vi "VisionTest.vi"() -> ()   [LabVIEW 2019]
uses:
  <vilib>/Analysis/coordinate.llb/2D Cartesian Coordinate Shift (Array).vi
  <vilib>/Analysis/coordinate.llb/2D Cartesian Coordinate Rotation (Array).vi
  <vilib>/vision/NI_Vision_Development_Module.lvlib
  <vilib>/Analysis/NI_AALPro.lvlib
  KNRm_ReMi_OS6_436Motor.lvlibp
panel:
  out "100%?":bool
  in  "Range (Threshold 1)":cluster{"Lower value":sgl, "Upper value":sgl}={"Lower value"=0.0, "Upper value"=97.0}
  in  "BCG Values (Brightness 1)":T1={"Brightness"=14.920213, "Contrast"=75.893616, "Gamma"=0.54697555}
  in  "appended array":cluster{"X":dbl, "Y":dbl}[][](array[cluster])=[[{"X"=-47.53091149865394, "Y"=-51.61265055692628}, {"X"=-21.409316336691, "Y"=-52.40940259624713}, {"X"=7.531820971180464, "Y"=-50.24379818829546}, {"X"=34.723675975177635, "Y"=-49.29998044211228}, {"X"=62.50311529948201, "Y"=-48.069245788503636}], [{"X"=-52.10358780846479, "Y"=-23.573317003903952}, {"X"=-23.218349773016104, "Y"=-21.445937136105403}, {"X"=5.683945770158462, "Y"=-22.15858586504581}, {"X"=35.18585318767401, "Y"=-19.06306176014282}, {"X"=66.71847272117144, "Y"=-21.228561633901943}], [{"X"=-51.985118485666646, "Y"=6.629238139360316}, {"X"=-24.25833990412113, "Y"=12.579982375452046}, {"X"=5.656895686551195, "Y"=6.522155781007332}, {"X"=35.67862718864419, "Y"=7.798470020464374}, {"X"=69.44473388807687, "Y"=0.3684014734527225}], [{"X"=-54.7434454883762, "Y"=29.606207620157388}, {"X"=-24.38816628097914, "Y"=37.122414150924804}, {"X"=4.619057492645264, "Y"=32.696655394047305}, {"X"=35.01737200966194, "Y"=31.653332942710716}, {"X"=65.85863943682, "Y"=26.744342832725305}], [{"X"=-59.40958389987326, "Y"=69.68736705460744}, {"X"=-22.67716866450974, "Y"=68.0170935631974}, {"X"=9.882161579130868, "Y"=66.7477246147916}, {"X"=41.15360353471889, "Y"=62.8768714318752}, {"X"=71.97577084980611, "Y"=58.197728561186445}]]
  in  "appended array 3":cluster{dbl, dbl}[][](array[cluster])=[[{-50.0, -30.0}, {-20.0, -30.0}, {10.0, -30.0}, {40.0, -30.0}, {70.0, -30.0}], [{-50.0, 0.0}, {-20.0, 0.0}, {10.0, 0.0}, {40.0, 0.0}, {70.0, 0.0}], [{-50.0, 30.0}, {-20.0, 30.0}, {10.0, 30.0}, {40.0, 30.0}, {70.0, 30.0}], [{-50.0, 60.0}, {-20.0, 60.0}, {10.0, 60.0}, {40.0, 60.0}, {70.0, 60.0}], [{-50.0, 90.0}, {-20.0, 90.0}, {10.0, 90.0}, {40.0, 90.0}, {70.0, 90.0}]]
  out "Boolean array":bool[](array[boolean])
  out "y":dbl
  out "x":dbl
  out "stop":bool
  out "botton":bool
  in  "y":dbl=15.0 format="%#_13g"
  out "ColorDet Img":T2(plugin-control)
  out "G":u16
  out "B":u16
  out "Class":string
  out "output Brick (x, y, theta)":dbl[](array[numeric])
  in  "Grab":bool
  out "Particle Measurements (Real-World) (Particle Analysis 1)":dbl[][](array[numeric]) format="%.2f"
  out "Number of Matches":i32
  out "Cal Img":T2(plugin-control)
  out "Bin Img":T2(plugin-control)
  in  "Stop Button":bool
  # "r"
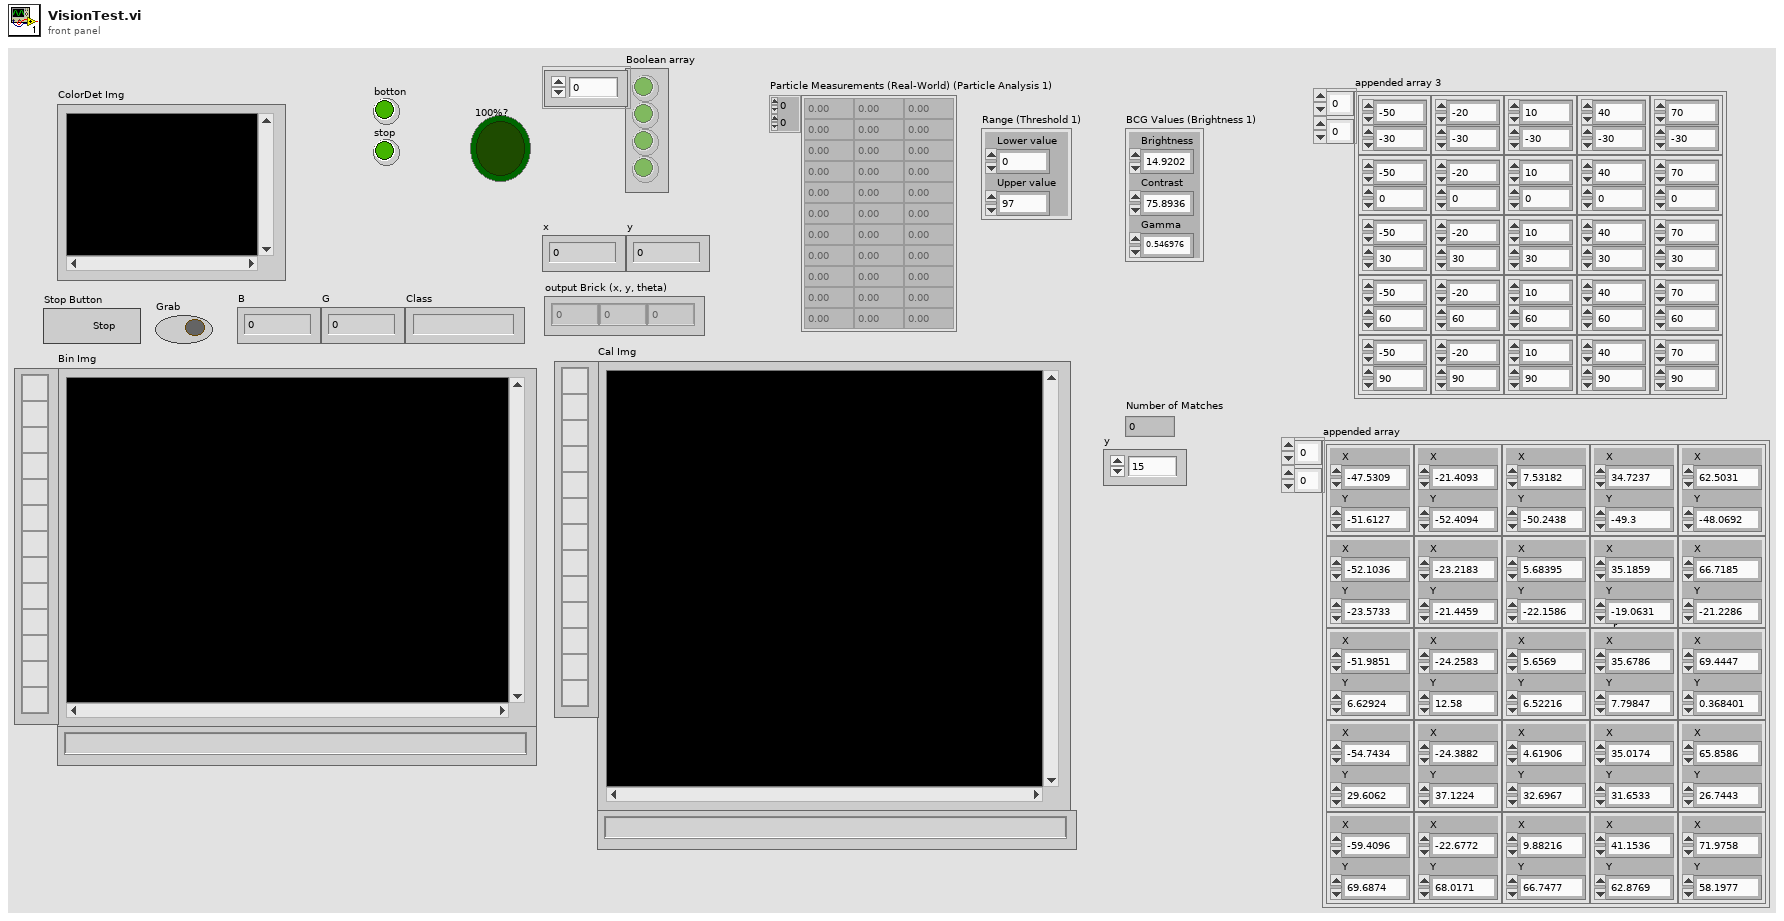
[diagram p1: front panel]
types:
  T1 = cluster{"Brightness":sgl, "Contrast":sgl, "Gamma":sgl}
  T2 = typedef "IMAQ Image.ctl" = refnum<image>
  T3 = typedef "Image Type" = u32
  T4 = cluster{"Interpolation Type":enum32{"Zero Order", "Bilinear", "Quadratic", "Cubic", "Bilinear Fixed"}, "Destination Width":u32, "Destination Height":u32, "Fill Value":sgl}
  T5 = cluster{"Particle Measurements (Real-World) (Particle Analysis 1)":dbl[], "Class":string}
  T6 = enum16{"P1", "P2", "P3", "P4", "P5", "P6", "OUT", "take a picture"}
  T7 = cluster{"Numeric":u8, "Numeric":u8, "Numeric":u8, "Numeric":u8}
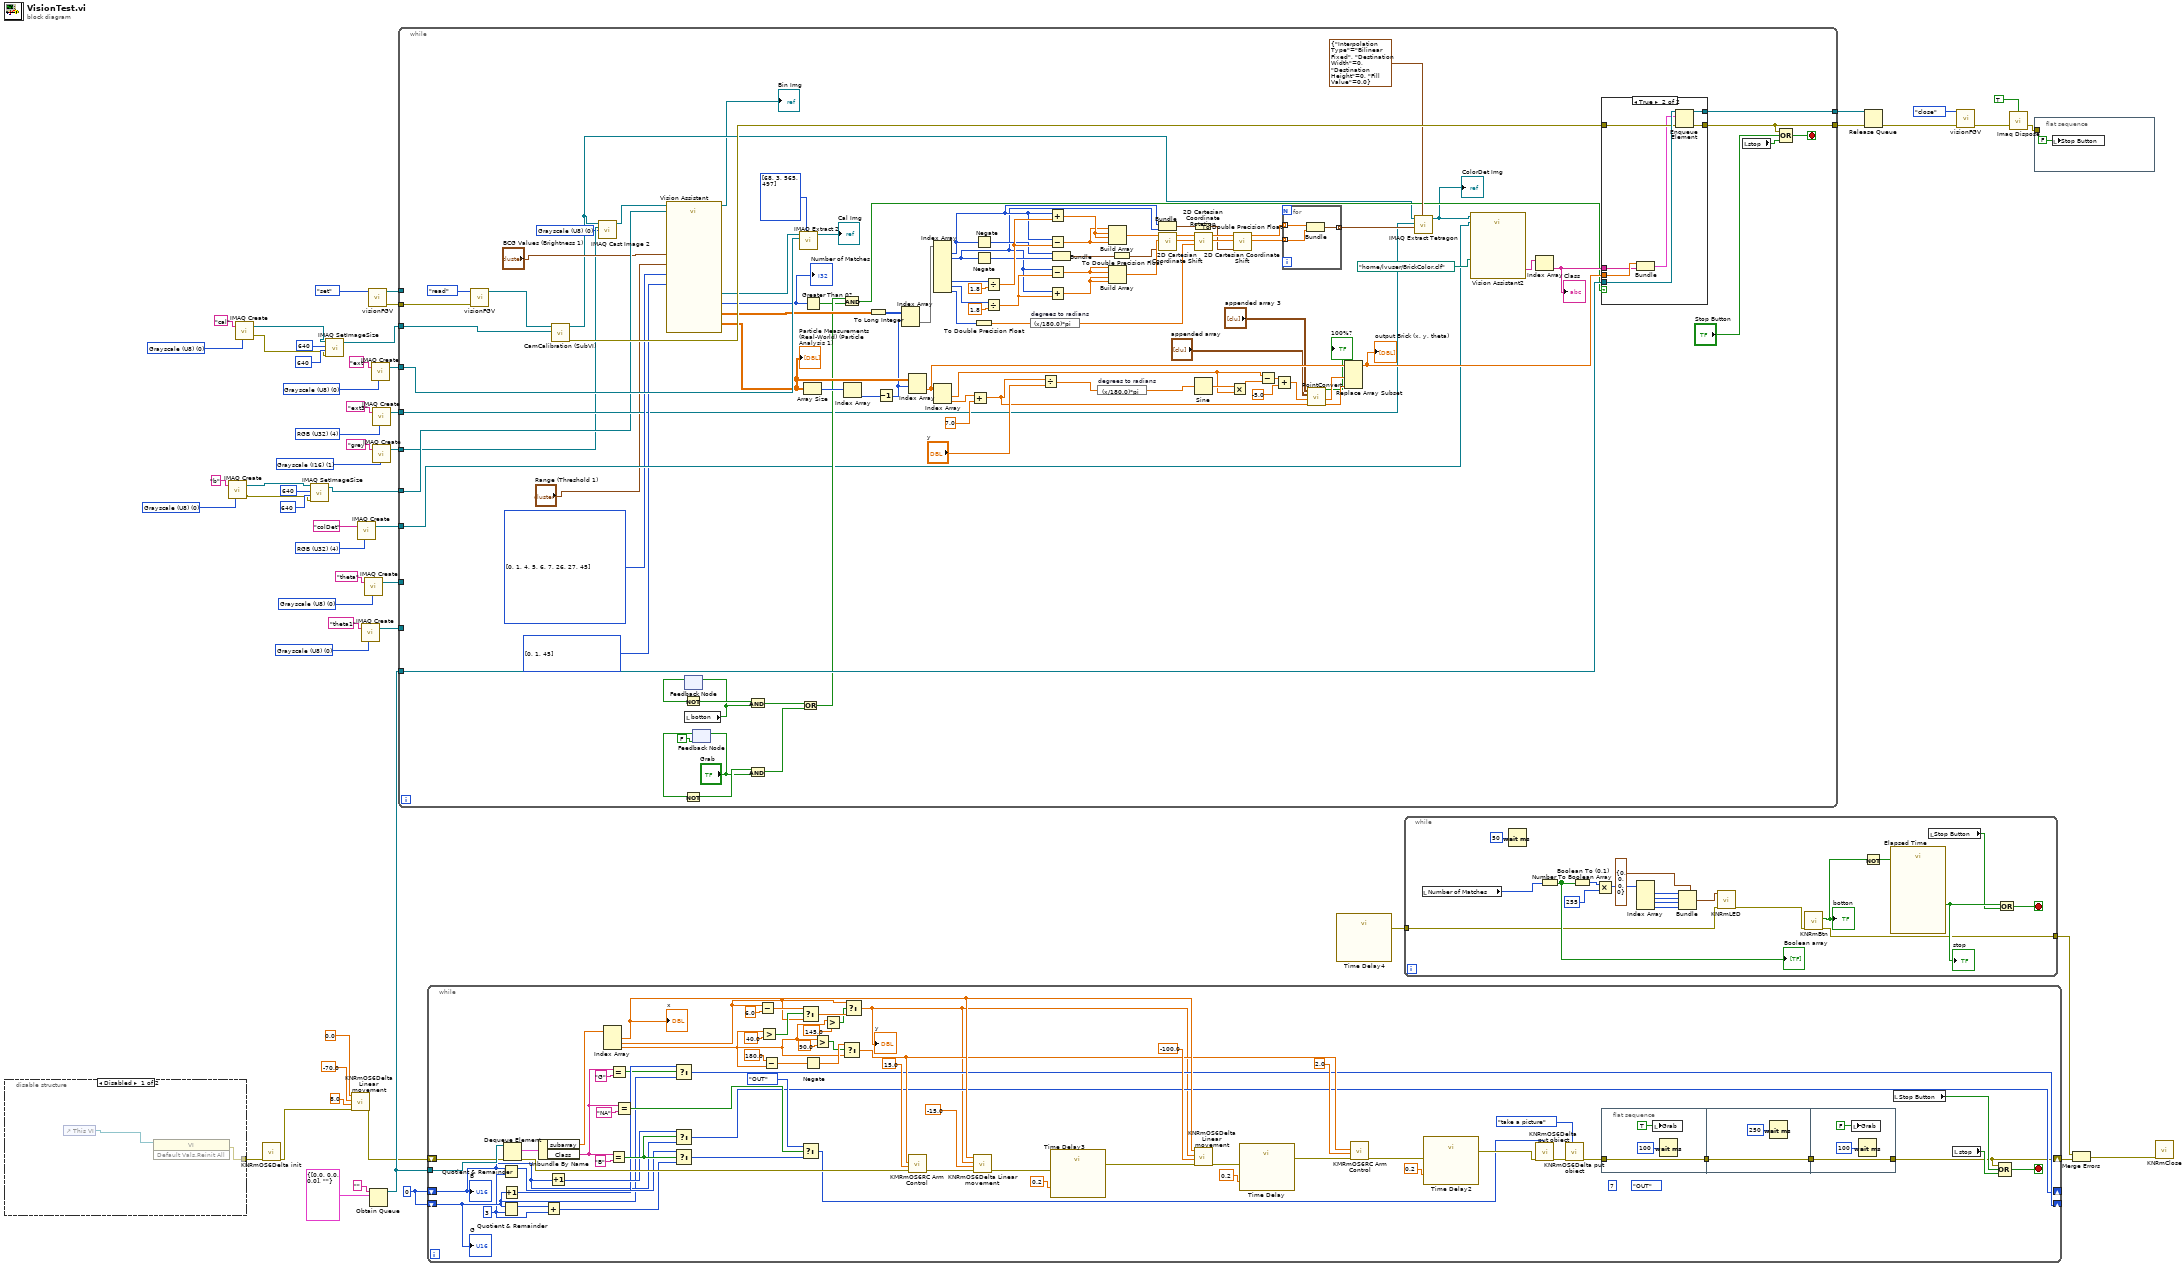
[diagram p0: block diagram]
diagram:
  w14 = T3 0 items=["Grayscale (U8)", "Grayscale (I16)", "Grayscale (SGL)", "Complex (CSG)", "RGB (U32)", "HSL (U32)", "RGB (U64)", "Grayscale (U16)"] ("Image Type")
  w24 = T3 0 items=["Grayscale (U8)", "Grayscale (I16)", "Grayscale (SGL)", "Complex (CSG)", "RGB (U32)", "HSL (U32)", "RGB (U64)", "Grayscale (U16)"] ("Image Type")
  w29 = T3 4 items=["Grayscale (U8)", "Grayscale (I16)", "Grayscale (SGL)", "Complex (CSG)", "RGB (U32)", "HSL (U32)", "RGB (U64)", "Grayscale (U16)"] ("Image Type")
  w31 = u16 0
  w34 = T3 4 items=["Grayscale (U8)", "Grayscale (I16)", "Grayscale (SGL)", "Complex (CSG)", "RGB (U32)", "HSL (U32)", "RGB (U64)", "Grayscale (U16)"] ("Image Type")
  w42 = T3 0 items=["Grayscale (U8)", "Grayscale (I16)", "Grayscale (SGL)", "Complex (CSG)", "RGB (U32)", "HSL (U32)", "RGB (U64)", "Grayscale (U16)"] ("Image Type")
  w45 = T3 0 items=["Grayscale (U8)", "Grayscale (I16)", "Grayscale (SGL)", "Complex (CSG)", "RGB (U32)", "HSL (U32)", "RGB (U64)", "Grayscale (U16)"] ("Image Type")
  w47 = T3 0 items=["Grayscale (U8)", "Grayscale (I16)", "Grayscale (SGL)", "Complex (CSG)", "RGB (U32)", "HSL (U32)", "RGB (U64)", "Grayscale (U16)"] ("Image Type")
  w49 = T3 1 items=["Grayscale (U8)", "Grayscale (I16)", "Grayscale (SGL)", "Complex (CSG)", "RGB (U32)", "HSL (U32)", "RGB (U64)", "Grayscale (U16)"] ("Image Type")
  n1 = disable-structure shown="Disabled" {
    disable-tunnel: [w57 _] -> w12
    frame Disabled {
      n2 = control-ref of="This VI"() -> (w58:refnum<vi>)
      n3 = invoke class="VI" method="Default Vals.Reinit All"(reference=w58) -> (error out=w57:errorcluster)  [unwired: 2 in, 2 out]
    }
    frame Enabled {
    }
  }
  n4 = call "IMAQ Create"("Image Name"="b", "Image Type"=w42) -> ("New Image"=w3:T2, "error out"=w2:errorcluster)  [unwired: 3 in]
  n5 = call "IMAQ Create"("Image Name"="cal", "Image Type"=w47) -> ("New Image"=w8:T2, "error out"=w7:errorcluster)  [unwired: 3 in]
  n6 = call "KNRmOS6Delta init.vi"("error in (no error)"=w12) -> ("error out"=w17:errorcluster)  [unwired: 10 in]
  n7 = call "IMAQ SetImageSize"("error in (no error)"=w2, "Y Resolution"=640, "X Resolution"=640, "Image"=w3) -> ("Image Out"=w1:T2)  [unwired: 1 in, 1 out]
  n8 = call "IMAQ SetImageSize"("error in (no error)"=w7, "Y Resolution"=640, "X Resolution"=640, "Image"=w8) -> ("Image Out"=w6:T2)  [unwired: 1 in, 1 out]
  n9 = call "KNRmOS6Delta Linear movement.vi"("error in (no error)"=w17, "z0"=8.0, "y0"=-70.0, "x0"=0.0) -> ("error out"=w16:errorcluster)  [unwired: 7 in]
  n10 = call "IMAQ Create"("Image Name"="colDet", "Image Type"=w34) -> ("New Image"=w33:T2)  [unwired: 3 in, 1 out]
  n11 = call "IMAQ Create"("Image Name"="theta1", "Image Type"=w14) -> ("New Image"=w13:T2)  [unwired: 3 in, 1 out]
  n12 = call "IMAQ Create"("Image Name"="theta", "Image Type"=w24) -> ("New Image"=w22:T2)  [unwired: 3 in, 1 out]
  n13 = call "visionFGV.vi"("Function"=enum16{"set", "read", "close"}."set") -> ("error out"=w51:errorcluster, "Image Out fgv"=w55:T2)  [unwired: 9 in]
  n14 = Obtain Queue(name (unnamed)="", element data type=cluster{"subarray":dbl[], "Class":string} {"subarray"=[0.0, 0.0, 0.0], "Class"=""}) -> (queue out=w39:refnum<queue>)  [unwired: 3 in, 2 out]
  n15 = call "IMAQ Create"("Image Name"="ext", "Image Type"=w45) -> ("New Image"=w44:T2)  [unwired: 3 in, 1 out]
  n16 = call "IMAQ Create"("Image Name"="ext3", "Image Type"=w29) -> ("New Image"=w28:T2)  [unwired: 3 in, 1 out]
  n17 = call "IMAQ Create"("Image Name"="grey", "Image Type"=w49) -> ("New Image"=w48:T2)  [unwired: 3 in, 1 out]
  n18 = while {
    tunnel: w55 -> [_]
    tunnel: w51 -> [w158]
    tunnel: w48 -> [w64]
    tunnel: w6 -> [w75]
    tunnel: w44 -> [w156]
    tunnel: w1 -> [w74]
    tunnel: w39 -> [w154]
    tunnel: [w98] -> w38
    tunnel: [w152] -> w36
    tunnel: w33 -> [w87]
    tunnel: w28 -> [w78]
    tunnel: w22 -> [_]
    tunnel: w13 -> [_]
    stop <- w95 stop-if-true
    w62 = T3 0 items=["Grayscale (U8)", "Grayscale (I16)", "Grayscale (SGL)", "Complex (CSG)", "RGB (U32)", "HSL (U32)", "RGB (U64)", "Grayscale (U16)"] ("Image Type")
    w81 = i32[] [0, 1, 4, 5, 6, 7, 26, 27, 45] items=["Center of Mass X", "Center of Mass Y", "First Pixel X", "First Pixel Y", "Bounding Rect Left", "Bounding Rect Top", "Bounding Rect Right", "Bounding Rect Bottom", "Max Feret Diameter Start X", "Max Feret Diameter Start Y", "Max Feret Diameter End X", "Max Feret Diameter End Y", "Max Horiz. Segment Length Left", "Max Horiz. Segment Length Right", "Max Horiz. Segment Length Row", "-", "Bounding Rect Width", "Bounding Rect Height", "Bounding Rect Diagonal", "Perimeter", "Convex Hull Perimeter", "Holes' Perimeter", "Max Feret Diameter", "Equivalent Ellipse Major Axis", "Equivalent Ellipse Minor Axis", "Equivalent Ellipse Minor Axis (Feret)", "Equivalent Rect Long Side", "Equivalent Rect Short Side", "Equivalent Rect Diagonal", "Equivalent Rect Short Side (Feret)", "Average Horiz. Segment Length", "Average Vert. Segment Length", "Hydraulic Radius", "Waddel Disk Diameter", "-", "Area", "Holes' Area", "Particle & Holes' Area", "Convex Hull Area", "Image Area", "-", "Number of Holes", "Number of Horiz. Segments", "Number of Vert. Segments", "-", "Orientation", "Max Feret Diameter Orientation", "-", "% Area/Image Area", "% Area/(Particle & Holes' Area)", "Ratio of Equivalent Ellipse Axes", "Ratio of Equivalent Rect Sides", "-", "Elongation Factor", "Compactness Factor", "Heywood Circularity Factor", "Type Factor", "-", "Sum X", "Sum Y", "Sum XX", "Sum XY", "Sum YY", "Sum XXX", "Sum XXY", "Sum XYY", "Sum YYY", "-", "Moment of Inertia XX", "Moment of Inertia XY", "Moment of Inertia YY", "Moment of Inertia XXX", "Moment of Inertia XXY", "Moment of Inertia XYY", "Moment of Inertia YYY", "Norm. Moment of Inertia XX", "Norm. Moment of Inertia XY", "Norm. Moment of Inertia YY", "Norm. Moment of Inertia XXX", "Norm. Moment of Inertia XXY", "Norm. Moment of Inertia XYY", "Norm. Moment of Inertia YYY", "Hu Moment 1", "Hu Moment 2", "Hu Moment 3", "Hu Moment 4", "Hu Moment 5", "Hu Moment 6", "Hu Moment 7"] ("Pixel Measurements (Particle Analysis 1)")
    w80 = i32[] [0, 1, 45] items=["Center of Mass X", "Center of Mass Y", "First Pixel X", "First Pixel Y", "Bounding Rect Left", "Bounding Rect Top", "Bounding Rect Right", "Bounding Rect Bottom", "Max Feret Diameter Start X", "Max Feret Diameter Start Y", "Max Feret Diameter End X", "Max Feret Diameter End Y", "Max Horiz. Segment Length Left", "Max Horiz. Segment Length Right", "Max Horiz. Segment Length Row", "-", "Bounding Rect Width", "Bounding Rect Height", "Bounding Rect Diagonal", "Perimeter", "Convex Hull Perimeter", "Holes' Perimeter", "Max Feret Diameter", "Equivalent Ellipse Major Axis", "Equivalent Ellipse Minor Axis", "Equivalent Ellipse Minor Axis (Feret)", "Equivalent Rect Long Side", "Equivalent Rect Short Side", "Equivalent Rect Diagonal", "Equivalent Rect Short Side (Feret)", "Average Horiz. Segment Length", "Average Vert. Segment Length", "Hydraulic Radius", "Waddel Disk Diameter", "-", "Area", "Holes' Area", "Particle & Holes' Area", "Convex Hull Area", "Image Area", "-", "Number of Holes", "Number of Horiz. Segments", "Number of Vert. Segments", "-", "Orientation", "Max Feret Diameter Orientation", "-", "% Area/Image Area", "% Area/(Particle & Holes' Area)", "Ratio of Equivalent Ellipse Axes", "Ratio of Equivalent Rect Sides", "-", "Elongation Factor", "Compactness Factor", "Heywood Circularity Factor", "Type Factor", "-", "Sum X", "Sum Y", "Sum XX", "Sum XY", "Sum YY", "Sum XXX", "Sum XXY", "Sum XYY", "Sum YYY", "-", "Moment of Inertia XX", "Moment of Inertia XY", "Moment of Inertia YY", "Moment of Inertia XXX", "Moment of Inertia XXY", "Moment of Inertia XYY", "Moment of Inertia YYY", "Norm. Moment of Inertia XX", "Norm. Moment of Inertia XY", "Norm. Moment of Inertia YY", "Norm. Moment of Inertia XXX", "Norm. Moment of Inertia XXY", "Norm. Moment of Inertia XYY", "Norm. Moment of Inertia YYY", "Hu Moment 1", "Hu Moment 2", "Hu Moment 3", "Hu Moment 4", "Hu Moment 5", "Hu Moment 6", "Hu Moment 7"] ("Real-World Measurements (Particle Analysis 1)")
    n19 = call "visionFGV.vi"("Error In"=w158, "Function"=enum16{"set", "read", "close"}."read") -> ("Image Out fgv"=w77:T2)  [unwired: 8 in, 1 out]
    n20 = call "CamCalibration (SubVI).vi"("Image Dst"=w75, "Image In"=w77) -> ("error out"=w153:errorcluster, "Image Out"=w63:T2)  [unwired: 8 in]
    n21 = call "IMAQ Cast Image 2"("Image Src"=w63, "Image Dst"=w64, "Image Type"=w62) -> ("Image Dst Out"=w61:T2)  [unwired: 11 in, 1 out]
    n22 = call "Vision Assistant"("Image In"=w61, "Image Dst"=w74, "BCG Values (Brightness 1)"="BCG Values (Brightness 1)", "Range (Threshold 1)"="Range (Threshold 1)", "Pixel Measurements (Particle Analysis 1)"=w81, "Real-World Measurements (Particle Analysis 1)"=w80) -> ("Image Out"=→"Bin Img":T2, "Number of Particles (Particle Analysis 1)"=w101:i32, "Particle Measurements (Real-World) (Particle Analysis 1)"=w147:dbl[][], "Particle Measurements (Pixels) (Particle Analysis 1)"=w139:dbl[][], "Image Buffer (Image Buffer 2)"=w145:T2)  [unwired: 16 in, 1 out]
    "Number of Matches" <- w101
    "Particle Measurements (Real-World) (Particle Analysis 1)" <- w147
    n23 = feedback #1() -> (w93:bool)  [unwired: 1 in]
    n24 = Not(x=w93) -> (.not. x?=w92:bool)
    n25 = local read "botton"() -> (w91:bool)
    n26 = feedback-in #1(w91) -> ()
    n27 = feedback-in #2("Grab") -> ()
    n28 = feedback #2(FALSE ("Grab")) -> (w151:bool)
    n29 = Not(x=w151) -> (.not. x?=w150:bool)
    n30 = And(x=w92, y=w91) -> (x .and. y?=w90:bool)
    n31 = And(x=w150, y="Grab") -> (x .and. y?=w103:bool)
    n32 = call "IMAQ Extract 2"("Optional Rectangle"=i32[] [68, 3, 565, 497] ("Global Rectangle"), "Image Dst"=w156, "Image Src"=w145) -> ("Image Dst Out"=→"Cal Img":T2)  [unwired: 7 in, 1 out]
    n33 = Or(x=w90, y=w103) -> (x .or. y?=w102:bool)
    n34 = Array Size(array=w147) -> (size(s)=w148:i32[])
    n35 = Greater Than 0?(x=w101) -> (x > 0?=w100:bool)
    n36 = And(x=w102, y=w100) -> (x .and. y?=w99:bool)
    n37 = Index Array(array=w148) -> (element=w146:i32)  [unwired: 1 in]
    n38 = To Long Integer(number=w139) -> (32bit integer=w138:i32[][])
    n39 = Decrement(x=w146) -> (x-1=w79:i32)
    n40 = Index Array(array=w138, index (row)=w79) -> (element=w76:i32[])  [unwired: 1 in]
    n41 = Index Array(array=w147, index (row)=w79) -> (element=w141:dbl[])  [unwired: 1 in]
    n42 = Index Array(array=w76) -> (element #1=w119:i32, element #2=w118:i32, element #7=w129:i32, element #8=w125:i32, element #9=w132:i32)  [unwired: 9 in, 4 out]
    n43 = Index Array(array=w141) -> (element #1=w69:dbl, element #2=w83:dbl)  [unwired: 2 in]
    n44 = Add(x=w83, y=7.0) -> (x+y=w73:dbl)
    n45 = Negate(x=w119) -> (-x=w121:i32)
    n46 = Negate(x=w118) -> (-x=w122:i32)
    n47 = To Double Precision Float(number=w132) -> (double precision float=w123:dbl)
    n48 = Divide(x=w129, y=1.8) -> (x/y=w127:dbl)
    n49 = Divide(x=w125, y=1.8) -> (x/y=w124:dbl)
    n50 = expression code="(x/180.0)*pi" "degrees to radians"(w123) -> (w131:dbl)
    n51 = Divide(x=w73, y="y") -> (x/y=w143:dbl)
    n52 = Add(x=w119, y=w127) -> (x+y=w136:dbl)
    n53 = Subtract(x=w119, y=w127) -> (x-y=w135:dbl)
    n54 = Subtract(x=w118, y=w124) -> (x-y=w134:dbl)
    n55 = Add(x=w118, y=w124) -> (x+y=w133:dbl)
    n56 = Bundle(w121, w122) -> (w120:cluster{i32, i32})  [unwired: 1 in]
    n57 = expression code="(x/180.0)*pi" "degrees to radians"(w143) -> (w108:dbl)
    n58 = Build Array(w135, w136, w136, w135) -> (w117:dbl[])
    n59 = Build Array(w134, w134, w133, w133) -> (w116:dbl[])
    n60 = To Double Precision Float(number=w120) -> (double precision float=w106:cluster{dbl, dbl})
    n61 = Bundle("Numeric"=w119, "Numeric"=w118) -> (w111:cluster{"Numeric":i32, "Numeric":i32})  [unwired: 1 in]
    n62 = call-poly <vilib>:"2D Cartesian Coordinate Shift.vi"("shift"=w106, "Y"=w116, "X"=w117) -> ("Y Out"=w114:dbl[], "X Out"=w115:dbl[])  [unwired: 6 in, 1 out]
    n63 = To Double Precision Float(number=w111) -> (double precision float=w107:cluster{"Numeric":dbl, "Numeric":dbl})
    n64 = call-poly <vilib>:"2D Cartesian Coordinate Rotation.vi"("theta"=w131, "Y"=w114, "X"=w115) -> ("Y Out"=w112:dbl[], "X Out"=w113:dbl[])  [unwired: 6 in, 1 out]
    n65 = Sine(x=w108) -> (sin(x)=w105:dbl)
    n66 = Multiply(x=w105, y=w69) -> (x*y=w142:dbl)
    n67 = call-poly <vilib>:"2D Cartesian Coordinate Shift.vi"("shift"=w107, "Y"=w112, "X"=w113) -> ("Y Out"=w109:dbl[], "X Out"=w110:dbl[])  [unwired: 6 in, 1 out]
    n68 = Subtract(x=w69, y=w142) -> (x-y=w85:dbl)
    n69 = Add(x=w85, y=-5.0) -> (x+y=w70:dbl)
    n70 = for {
      tunnel: w110 -> [w162] mode=indexing
      tunnel: w109 -> [w161] mode=indexing
      tunnel: [w160] -> w130 mode=indexing
      n71 = Bundle("Numeric"=w162, "Numeric"=w161) -> (w160:cluster{"Numeric":dbl, "Numeric":dbl})  [unwired: 1 in]
    }
    n72 = call "PointConvert.vi"("RealWorldY"=w73, "RealWorldX"=w70, "RealWorldXY"="appended array", "DeltaXY"="appended array 3") -> ("DeltaY"=w71:dbl, "DeltaX"=w72:dbl, "100%?"=→"100%?":bool)  [unwired: 5 in]
    n73 = Replace Array Subset(array=w141, new element #1=w72, new element #2=w71) -> (w140:dbl[])  [unwired: 2 in]
    "output Brick (x, y, theta)" <- w140
    n74 = call-poly "IMAQ Extract Tetragon"("Options"=T4 {"Interpolation Type"=enum."Bilinear Fixed", "Destination Width"=0, "Destination Height"=0, "Fill Value"=0.0}, "Tetragon"=w130, "Image Dst"=w78, "Image Src"=w63) -> ("Image Dst Out"=w88:T2)  [unwired: 6 in, 1 out]
    "ColorDet Img" <- w88
    n75 = call "Vision Assistant2"("Image In"=w88, "Image Dst"=w87, "File Path (Color Classification 1)"=path "/home/lvuser/BrickColor.clf") -> ("Classes (Color Classification 1)"=w86:string[])  [unwired: 22 in, 2 out]
    n76 = Index Array(array=w86) -> (element=w104:string)  [unwired: 1 in]
    "Class" <- w104
    n77 = case shown="True" w99 {
      tunnel: w154 -> [w163 w171]
      tunnel: w140 -> [_ w167]
      tunnel: [w164 w170] -> w98
      tunnel: w153 -> [w164 w169]
      tunnel: [w163 w168] -> w152
      tunnel: w104 -> [_ w166]
      frame False {
      }
      frame True {
        n78 = Bundle("Particle Measurements (Real-World) (Particle Analysis 1)"=w167, "Class"=w166) -> (w165:T5)  [unwired: 1 in]
        n79 = Enqueue Element(queue=w171, element=w165, error in (no error)=w169) -> (queue out=w168:refnum<queue>, error out=w170:errorcluster)  [unwired: 1 in, 1 out]
      }
    }
    n80 = local read "stop"() -> (w96:bool)
    n81 = Compound Arithmetic op=OR(w98, "Stop Button", w96) -> (w95:bool)
  }
  n82 = while {
    tunnel: w39 -> [w236]
    shift-right: [w177] -> w26
    shift-left: w16 -> [w228]
    shift-right: [w200] -> _
    shift-left: w31 -> [w199]
    shift-right: [w201] -> _
    shift-left: w31 -> [w198]
    stop <- w182 stop-if-true
    w196 = u16 3 ("y")
    (unwired) T6."OUT" ("move to")
    (unwired) 7 ("y")
    n83 = Quotient & Remainder(x=w199, y=w196) -> (x-y*floor(x/y)=w206:u16)  [unwired: 1 out]
    n84 = Increment(x=w198) -> (x+1=w205:u16)
    n85 = Quotient & Remainder(x=w198, y=w196) -> (x-y*floor(x/y)=w197:u16)  [unwired: 1 out]
    n86 = Dequeue Element(queue=w236, error in (no error)=w228) -> (element=w214:cluster{"subarray":dbl[], "Class":string}, error out=w232:errorcluster)  [unwired: 1 in, 2 out]
    n87 = Unbundle By Name(w214) -> ("subarray"=w213:dbl[], "Class"=w203:string)
    n88 = Add(x=w197, y=w196) -> (x+y=w195:u16)
    n89 = Increment(x=w199) -> (x+1=w207:u16)
    n90 = Index Array(array=w213) -> (element #1=w223:dbl, element #2=w185:dbl, element #3=w174:dbl)  [unwired: 3 in]
    "x" <- w223
    n91 = Equal?(x=w203, y="B") -> (x = y?=w208:bool)
    n92 = Equal?(x=w203, y="G") -> (x = y?=w202:bool)
    n93 = Equal?(x=w203, y="NA") -> (x = y?=w211:bool)
    n94 = Select(t=w205, s=w202, f=w198) -> (s? t:f=w201:u16)
    n95 = Select(t=w207, s=w208, f=w199) -> (s? t:f=w200:u16)
    n96 = Select(t=w206, s=w208, f=w195) -> (s? t:f=w194:u16)
    n97 = Subtract(x=w185, y=6.0 ("y 2")) -> (x-y=w187:dbl)
    n98 = Greater?(x=w174, y=40.0) -> (0:w188:bool)
    n99 = Subtract(x=180.0, y=w174) -> (x-y=w216:dbl)
    n100 = Select(t=w187, s=w188, f=w185) -> (s? t:f=w186:dbl)
    n101 = Select(t=T6."OUT" ("move to"), s=w211, f=w194) -> (s? t:f=w193:u16)
    n102 = Negate(x=w216) -> (-x=w215:dbl)
    n103 = Greater?(x=w174, y=90.0) -> (0:w192:bool)
    n104 = Greater?(x=w174, y=145.0) -> (0:w172:bool)
    n105 = Select(t=w215, s=w192, f=w174) -> (s? t:f=w217:dbl)
    n106 = Select(t=w185, s=w172, f=w186) -> (s? t:f=w190:dbl)
    "y" <- w190
    n107 = call "KMRmOS6RC Arm Control.vi"("error in (no error)"=w232, "clip"=15.0, "turn"=w217) -> ("error out"=w233:errorcluster)  [unwired: 6 in, 2 out]
    n108 = call "KNRmOS6Delta Linear movement.vi"("error in (no error)"=w233, "z0"=-15.0, "y0"=w190, "x0"=w223) -> ("error out"=w181:errorcluster)  [unwired: 7 in]
    n109 = call "Time Delay3"("error in (no error)"=w181, "Delay Time (s)"=0.2) -> ("error out"=w179:errorcluster)  [unwired: 9 in]
    n110 = call "KNRmOS6Delta Linear movement.vi"("error in (no error)"=w179, "z0"=-100.0, "y0"=w190, "x0"=w223) -> ("error out"=w224:errorcluster)  [unwired: 7 in]
    n111 = call "Time Delay"("error in (no error)"=w224, "Delay Time (s)"=0.2) -> ("error out"=w226:errorcluster)  [unwired: 9 in]
    n112 = call "KMRmOS6RC Arm Control.vi"("error in (no error)"=w226, "clip"=2.0, "turn"=w217) -> ("error out"=w222:errorcluster)  [unwired: 6 in, 2 out]
    n113 = call "Time Delay2"("error in (no error)"=w222, "Delay Time (s)"=0.2) -> ("error out"=w221:errorcluster)  [unwired: 9 in]
    n114 = call "KNRmOS6Delta put obiect.vi"("move to"=w193, "error in (no error)"=w221) -> ("error in (no error) 2"=w230:errorcluster)  [unwired: 9 in]
    n115 = call "KNRmOS6Delta put obiect.vi"("move to"=T6."take a picture", "error in (no error)"=w230) -> ("error in (no error) 2"=w178:errorcluster)  [unwired: 9 in]
    n116 = flat-sequence {
      tunnel: w178 -> [w239]
      tunnel: [w239] -> w175
      tunnel: [w240] -> w176
      tunnel: w175 -> [w240]
      tunnel: [w243] -> w177
      tunnel: w176 -> [w243]
      frame #0 {
        n117 = local write "Grab"(TRUE ("Grab")) -> ()
        n118 = Wait (ms)(milliseconds to wait=u32 100) -> ()  [unwired: 1 out]
      }
      frame #1 {
        n119 = Wait (ms)(milliseconds to wait=u32 250) -> ()  [unwired: 1 out]
      }
      frame #2 {
        n120 = local write "Grab"(FALSE ("Grab")) -> ()
        n121 = Wait (ms)(milliseconds to wait=u32 100) -> ()  [unwired: 1 out]
      }
    }
    n122 = local read "Stop Button"() -> (w184:bool)
    n123 = local read "stop"() -> (w183:bool)
    n124 = Compound Arithmetic op=OR(w177, w184, w183) -> (w182:bool)
    "B" <- w199
    "G" <- w198
  }
  n125 = call "Time Delay4"() -> ("error out"=w25:errorcluster)  [unwired: 11 in]
  n126 = while {
    tunnel: [w259] -> w27
    tunnel: w25 -> [w245]
    stop <- w262 stop-if-true
    n127 = local read "Number of Matches"() -> (w247:i32)
    n128 = Wait (ms)(milliseconds to wait=u32 50) -> ()  [unwired: 1 out]
    n129 = Number To Boolean Array(number=w247) -> (Boolean array=w246:bool[])
    "Boolean array" <- w246
    n130 = Boolean To (0,1)(Boolean=w246) -> (0, 1=w255:i16[])
    n131 = Multiply(x=w255, y=255) -> (x*y=w254:i32[])
    n132 = Index Array(array=w254) -> (element #1=w252:i32, element #2=w251:i32, element #3=w250:i32, element #4=w249:i32)  [unwired: 4 in]
    n133 = Bundle(cluster=T7 {"Numeric"=0, "Numeric"=0, "Numeric"=0, "Numeric"=0} ("LEDSet"), "Numeric"=w252, "Numeric"=w251, "Numeric"=w250, "Numeric"=w249) -> (w256:T7)
    n134 = call "KNRmLED.vi"("error in"=w245, "LEDSet"=w256) -> ("error out"=w248:errorcluster)  [unwired: 9 in]
    n135 = call "KNRmBtn.vi"("error in"=w248) -> ("error out"=w259:errorcluster, "myRIOButton"=w258:bool)  [unwired: 9 in]
    "botton" <- w258
    n136 = Not(x=w258) -> (.not. x?=w261:bool)
    n137 = call "Elapsed Time"("Reset"=w261) -> ("Time has Elapsed"=w264:bool)  [unwired: 11 in, 7 out]
    "stop" <- w264
    n138 = local read "Stop Button"() -> (w263:bool)
    n139 = Or(x=w264, y=w263) -> (x .or. y?=w262:bool)
  }
  n140 = Release Queue(queue=w36, error in (no error)=w38) -> (error out=w37:errorcluster)  [unwired: 1 in, 2 out]
  n141 = call "visionFGV.vi"("Error In"=w37, "Function"=enum16{"set", "read", "close"}."close") -> ("error out"=w52:errorcluster)  [unwired: 8 in, 1 out]
  n142 = call "Imaq Dispose"("All Images? (No)"=TRUE, "error in (no error)"=w52) -> ("error out"=w11:errorcluster)  [unwired: 4 in]
  n143 = flat-sequence {
    tunnel: w11 -> [_]
    frame #0 {
      n144 = local write "Stop Button"(FALSE ("Stop Button")) -> ()
    }
  }
  n145 = Merge Errors(w27, w26) -> (w21:errorcluster)
  n146 = call "KNRmClose.vi"("error in"=w21) -> ()  [unwired: 10 in, 1 out]
